vi "Facade.vi"(0 "Data In":T5, 2 "Display State In":T2, 3 "Container State":T4) -> (6 "Data Out":T5, 7 "Display State Out":T2, 8 "Action":T1)   [LabVIEW 2020, in "Input Criterion.xctl"]
uses:
  Input Criterion.xctl
  Data.vi
  Digital Input VIs/Tosca-Input Criterion.ctl
  epl-vi-lib/Utility VIs/Type Defs/Logic State.ctl
  <vilib>/_xctls/Container State.ctl
  State.vi
  Events.ctl
  Event Type.ctl
  Operator.vi
  <vilib>/_xctls/Action.ctl
  <vilib>/_xctls/XControlSupport.lvlib
panel:
  in  "Time":dbl caption="ms"
  in  "Operator":u16(ring) items=["", "AND", "OR"]
  in  "State":u16(ring) caption="for" items=["Low", "High", "Rising", "Falling"]
  in  "Name":u16(ring) caption="is"
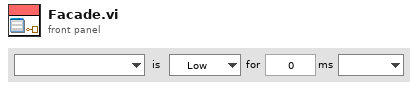
[diagram p1: front panel]
types:
  T1 = typedef "XControlSupport.lvlib/Action.ctl" = cluster{"Data Changed?":bool, "State Changed?":bool, "Action Name":string}
  T2 = typedef "Input Criterion.xctl/State.vi" = cluster{"DI":string[], "Flags":string[], "show op":bool, "flag start":i16, "Events":T3}
  T3 = typedef "Input Criterion.xctl/Events.ctl" = cluster{"Generic":refnum<user-event>, "Operator":refnum<user-event>, "Criterion":refnum<user-event>}
  T4 = typedef "XControlSupport.lvlib/Container State.ctl" = cluster{"Indicator?":bool, "Run Mode?":bool, " Refnum":refnum<vi>}
  T5 = typedef "Input Criterion.xctl/Data.vi" = cluster{"Criterion":T6, "Operator":i16, "visible":bool}
  T6 = typedef "Tosca-Input Criterion.ctl" = cluster{"DigInput":i32, "State":T7, "Time (ms)":i32, "Name":string}
  T7 = typedef "Logic State.ctl" = enum16{"Low", "High", "Rising", "Falling"}
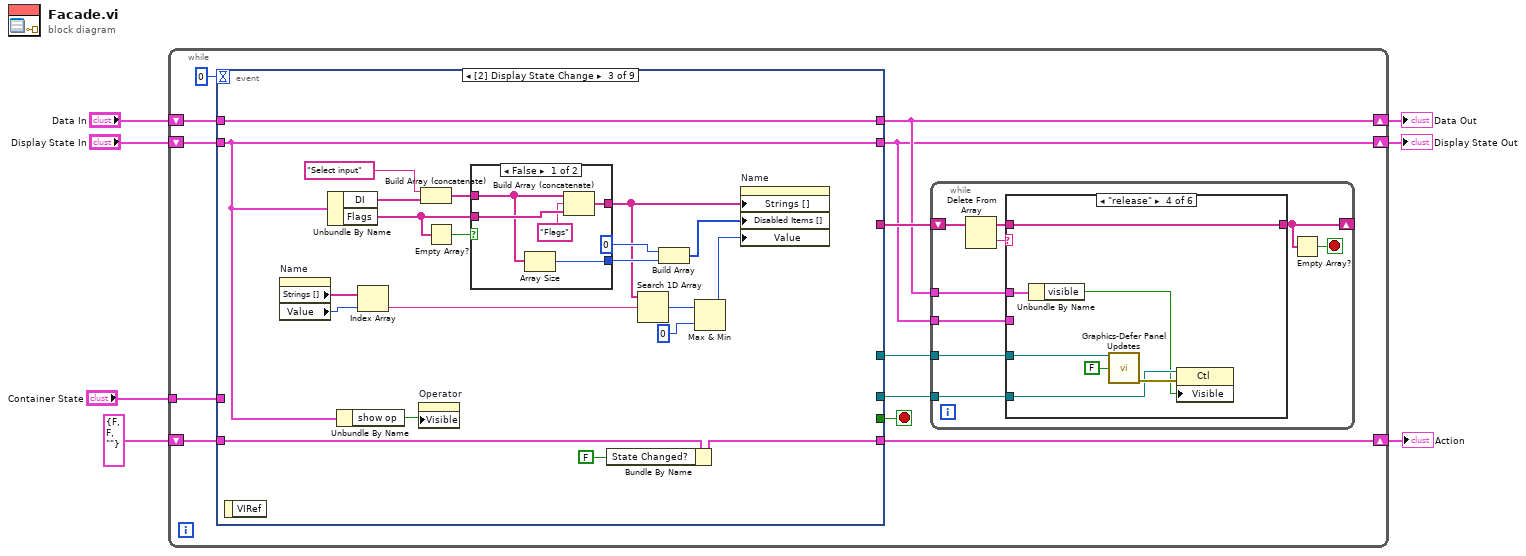
[diagram p0: block diagram]
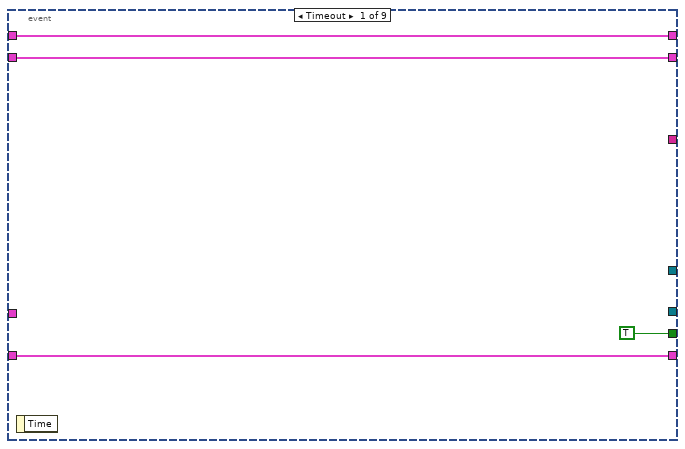
[diagram p2: hidden frame]
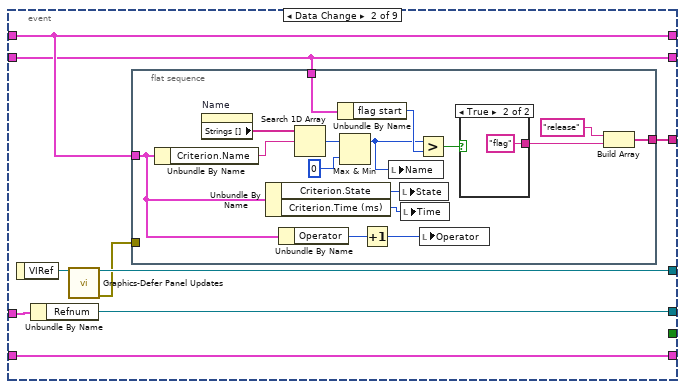
[diagram p3: hidden frame]
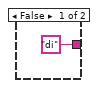
[diagram p4: hidden frame]
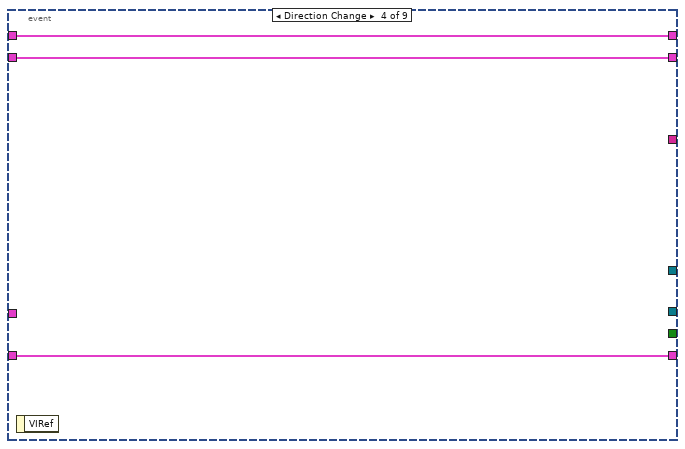
[diagram p6: hidden frame]
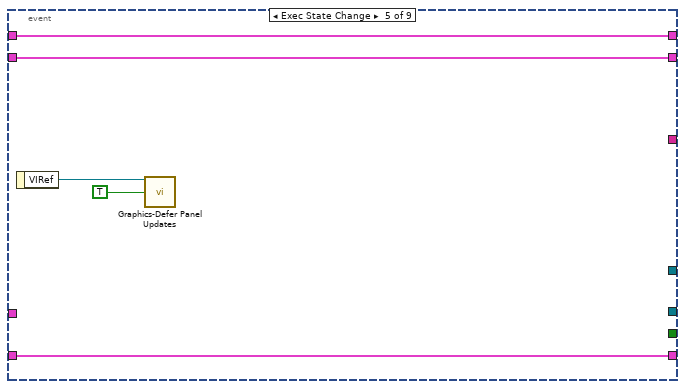
[diagram p7: hidden frame]
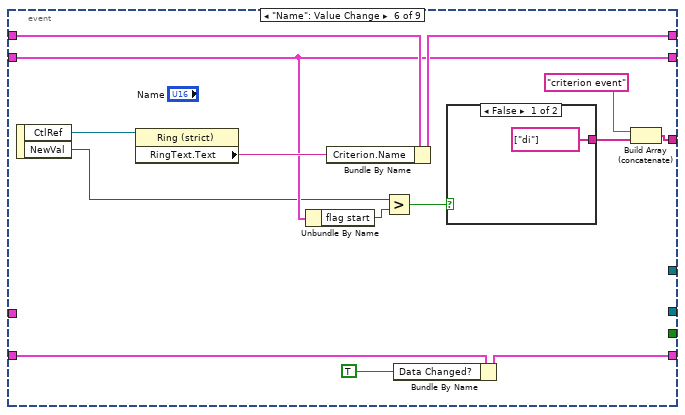
[diagram p8: hidden frame]
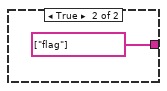
[diagram p9: hidden frame]
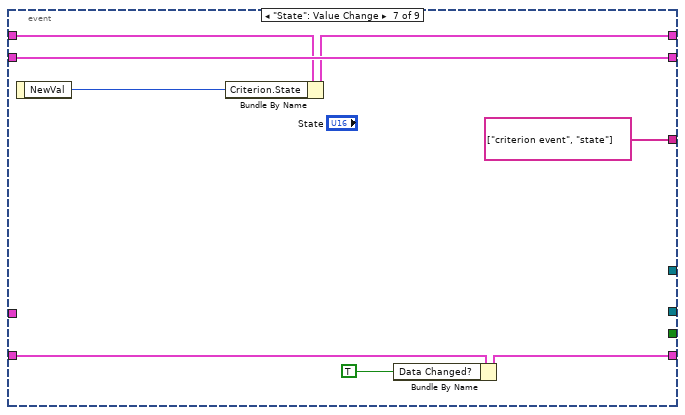
[diagram p10: hidden frame]
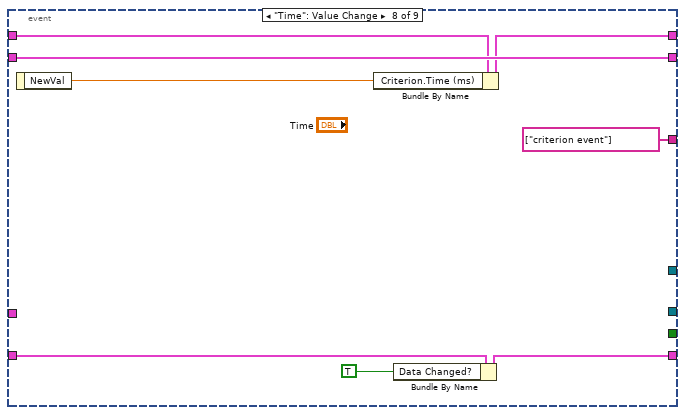
[diagram p11: hidden frame]
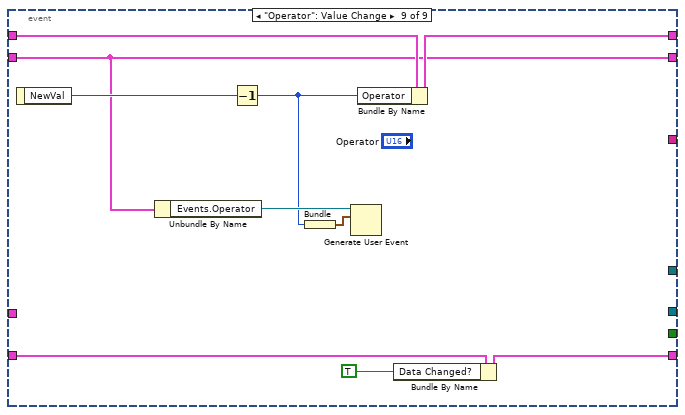
[diagram p12: hidden frame]
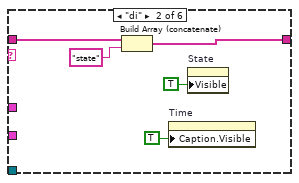
[diagram p14: hidden frame]
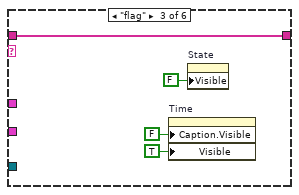
[diagram p15: hidden frame]
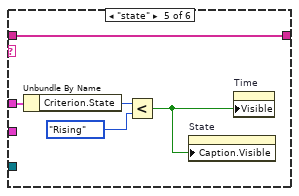
[diagram p16: hidden frame]
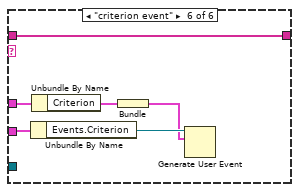
[diagram p17: hidden frame]
diagram:
  n1 = while {
    shift-right: [w9] -> w4
    shift-left: "Display State In" -> [w19]
    tunnel: "Container State" -> [w16]
    shift-right: [w11] -> w7
    shift-left: "Data In" -> [w15]
    shift-right: [w13] -> w2
    shift-left: T1 {"Data Changed?"=FALSE, "State Changed?"=FALSE, "Action Name"=""} ("Action") -> [w14]
    stop <- w18 stop-if-true
    n2 = event shown="[2] Display State Change" {
      selector: _ -> [_ _ _ _ _ _ _ _ _]
      dyn-events: _ -> [_ _ _ _ _ _ _ _ _]
      timeout: 0 -> [_ _ _ _ _ _ _ _ _]
      tunnel: w19 -> [w21 w30 w64 w80 w85 w91 w109 w117 w121]
      tunnel: [w21 w30 w64 w80 w85 w91 w109 w117 w121] -> w9
      tunnel: [TRUE _ _ _ _ _ _ _ _] -> w18
      tunnel: w16 -> [_ w25 _ _ _ _ _ _ _]
      tunnel: w15 -> [w20 w31 w71 w79 w84 w99 w108 w116 w127]
      tunnel: [w20 w31 w71 w79 w84 w94 w103 w112 w123] -> w11
      tunnel: [w22 w32 w60 w78 w83 w97 w106 w114 w125] -> w13
      tunnel: w14 -> [w22 w32 w70 w78 w83 w98 w107 w115 w126]
      tunnel: [_ w29 _ _ _ w87 string[] ["criterion event", "state"] string[] ["criterion event"] _] -> w12
      tunnel: [_ w27 _ _ _ _ _ _ _] -> w10
      tunnel: [_ w24 _ _ _ _ _ _ _] -> w8
      event Timeout {
        n3 = event-data() -> ()  [unwired: 1 in, 1 out]
      }
      event Data Change {
        n4 = event-data() -> ("VIRef"=w28:refnum<vi>)  [unwired: 1 in]
        n5 = Unbundle By Name(w25) -> ("Refnum"=w24:refnum<vi>)
        n6 = call "Graphics-Defer Panel Updates.vi"("VI"=w28) -> ("VI out"=w27:refnum<vi>, "error out"=w26:errorcluster)  [unwired: 13 in]
        n7 = flat-sequence {
          tunnel: w31 -> [w46]
          tunnel: w30 -> [w39]
          tunnel: [w34] -> w29
          tunnel: w26 -> [_]
          frame #0 {
            n8 = Unbundle By Name(w46) -> ("Criterion.Name"=w36:string)
            n9 = property on="Name" class="Ring (strict)"() -> ("Strings []"=w42:string[])  [unwired: 2 in, 2 out]
            n10 = Unbundle By Name(w46) -> ("Criterion.State"=w48:T7, "Criterion.Time (ms)"=w47:i32)
            n11 = Unbundle By Name(w46) -> ("Operator"=w45:i16)
            n12 = Search 1D Array(1D array=w42, element=w36) -> (index of element=w41:i32)  [unwired: 1 in]
            n13 = Unbundle By Name(w39) -> ("flag start"=w38:i16)
            n14 = Max & Min(x=w41, y=0) -> (max(x,y)=w35:i32)  [unwired: 1 out]
            n15 = Increment(x=w45) -> (x+1=w44:i16)
            n16 = local write "Name"(w35) -> ()
            n17 = local write "State"(w48) -> ()
            n18 = local write "Time"(w47) -> ()
            n19 = Greater?(x=w35, y=w38) -> (0:w37:bool)
            n20 = local write "Operator"(w44) -> ()
            n21 = case shown="True" w37 {
              tunnel: ["di" ("String") "flag" ("String")] -> w43
              frame False {
              }
              frame True {
              }
            }
            n22 = Build Array("release" ("element"), w43) -> (w34:string[])
          }
        }
      }
      event Display State Change {
        n23 = event-data() -> ()  [unwired: 1 in, 1 out]
        n24 = property on="Name" class="Ring (strict)"() -> ("Strings []"=w57:string[], "Value"=w56:u16)  [unwired: 2 in, 2 out]
        n25 = Unbundle By Name(w64) -> ("DI"=w69:string[], "Flags"=w65:string[])
        n26 = Unbundle By Name(w64) -> ("show op"=w63:bool)
        n27 = Index Array(array=w57, index=w56) -> (element=w54:string)
        n28 = property on="Operator" class="Ring (strict)"("Visible"=w63) -> ()  [unwired: 2 in, 2 out]
        n29 = Build Array (concatenate)("Select input", w69) -> (w67:string[])
        n30 = Empty Array?(array=w65) -> (empty?=w66:bool)
        n31 = case shown="False" w66 {
          tunnel: w67 -> [w73 w77]
          tunnel: w65 -> [w76 _]
          tunnel: [w74 w77] -> w55
          tunnel: [w72 _] -> w58
          frame False {
            n32 = Array Size(array=w73) -> (size(s)=w72:i32)
            n33 = Build Array (concatenate)(w73, "Flags", w76) -> (w74:string[])
          }
          frame True {
          }
        }
        n34 = Bundle By Name(cluster=w70, "State Changed?"=FALSE) -> (w60:T1)
        n35 = Search 1D Array(1D array=w55, element=w54) -> (index of element=w53:i32)  [unwired: 1 in]
        n36 = Build Array(0, w58) -> (w62:i32[])
        n37 = Max & Min(x=w53, y=0) -> (max(x,y)=w52:i32)  [unwired: 1 out]
        n38 = property on="Name" class="Ring (strict)"("Strings []"=w55, "Disabled Items []"=w62, "Value"=w52) -> ()  [unwired: 2 in, 2 out]
      }
      event Direction Change {
        n39 = event-data() -> ()  [unwired: 1 in, 1 out]
      }
      event Exec State Change {
        n40 = event-data() -> ("VIRef"=w82:refnum<vi>)  [unwired: 1 in]
        n41 = call "Graphics-Defer Panel Updates.vi"("VI"=w82, "Defer (F)"=TRUE) -> ()  [unwired: 12 in, 2 out]
      }
      event "Name": Value Change {
        n42 = event-data() -> ("CtlRef"=w93:refnum<vi>, "NewVal"=w90:u16)  [unwired: 1 in]
        n43 = property class="Ring (strict)"(reference=w93) -> ("RingText.Text"=w92:string)  [unwired: 1 in, 2 out]
        n44 = Unbundle By Name(w91) -> ("flag start"=w89:i16)
        n45 = Bundle By Name(cluster=w99, "Criterion.Name"=w92) -> (w94:T5)
        n46 = Greater?(x=w90, y=w89) -> (0:w88:bool)
        n47 = Bundle By Name(cluster=w98, "Data Changed?"=TRUE) -> (w97:T1)
        n48 = case shown="False" w88 {
          tunnel: [string[] ["di"] string[] ["flag"]] -> w95
          frame False {
          }
          frame True {
          }
        }
        n49 = Build Array (concatenate)("criterion event", w95) -> (w87:string[])
      }
      event "State": Value Change {
        n50 = event-data() -> ("NewVal"=w102:u16)  [unwired: 1 in]
        n51 = Bundle By Name(cluster=w108, "Criterion.State"=w102) -> (w103:T5)
        n52 = Bundle By Name(cluster=w107, "Data Changed?"=TRUE) -> (w106:T1)
      }
      event "Time": Value Change {
        n53 = event-data() -> ("NewVal"=w111:dbl)  [unwired: 1 in]
        n54 = Bundle By Name(cluster=w116, "Criterion.Time (ms)"=w111) -> (w112:T5)
        n55 = Bundle By Name(cluster=w115, "Data Changed?"=TRUE) -> (w114:T1)
      }
      event "Operator": Value Change {
        n56 = event-data() -> ("NewVal"=w122:u16)  [unwired: 1 in]
        n57 = Unbundle By Name(w121) -> ("Events.Operator"=w120:refnum<user-event>)
        n58 = Decrement(x=w122) -> (x-1=w119:u16)
        n59 = Bundle(w119) -> (w118:cluster{u16})  [unwired: 1 in]
        n60 = Generate User Event(user event=w120, event data cluster=w118) -> ()  [unwired: 2 in, 2 out]
        n61 = Bundle By Name(cluster=w127, "Operator"=w119) -> (w123:T5)
        n62 = Bundle By Name(cluster=w126, "Data Changed?"=TRUE) -> (w125:T1)
      }
    }
    n63 = while {
      shift-right: [w133] -> _
      shift-left: w12 -> [w136]
      tunnel: w11 -> [w131]
      tunnel: w10 -> [w130]
      tunnel: w9 -> [w129]
      tunnel: w8 -> [w128]
      stop <- w132 stop-if-true
      n64 = Delete From Array(array=w136) -> (deleted portion=w134:string, array with subset deleted=w135:string[])  [unwired: 2 in]
      n65 = case shown="\"release\"" w134 {
        tunnel: w135 -> [w137 w142 w146 w153 w158 w164]
        tunnel: [w137 w139 w146 w153 w158 w164] -> w133
        tunnel: w131 -> [_ _ _ w148 w157 w162]
        tunnel: w130 -> [_ _ _ w151 _ _]
        tunnel: w129 -> [_ _ _ _ _ w163]
        tunnel: w128 -> [_ _ _ w149 _ _]
        frame "", Default {
        }
        frame "di" {
          n66 = Build Array (concatenate)(w142, "state") -> (w139:string[])
          n67 = property on="Time" class="DigNum (strict)"("Caption.Visible"=TRUE) -> ()  [unwired: 2 in, 2 out]
          n68 = property on="State" class="Ring (strict)"("Visible"=TRUE) -> ()  [unwired: 2 in, 2 out]
        }
        frame "flag" {
          n69 = property on="Time" class="DigNum (strict)"("Caption.Visible"=FALSE, "Visible"=TRUE) -> ()  [unwired: 2 in, 2 out]
          n70 = property on="State" class="Ring (strict)"("Visible"=FALSE) -> ()  [unwired: 2 in, 2 out]
        }
        frame "release" {
          n71 = Unbundle By Name(w148) -> ("visible"=w147:bool)
          n72 = call "Graphics-Defer Panel Updates.vi"("VI"=w151, "Defer (F)"=FALSE) -> ("error out"=w150:errorcluster)  [unwired: 12 in, 1 out]
          n73 = property class="Ctl"(reference=w149, error in=w150, "Visible"=w147) -> ()  [unwired: 2 out]
        }
        frame "state" {
          n74 = Unbundle By Name(w157) -> ("Criterion.State"=w156:T7)
          n75 = Less?(x=w156, y=Logic_State."Rising") -> (x < y?=w154:bool)
          n76 = property on="State" class="Ring (strict)"("Caption.Visible"=w154) -> ()  [unwired: 2 in, 2 out]
          n77 = property on="Time" class="DigNum (strict)"("Visible"=w154) -> ()  [unwired: 2 in, 2 out]
        }
        frame "criterion event" {
          n78 = Unbundle By Name(w163) -> ("Events.Criterion"=w160:refnum<user-event>)
          n79 = Unbundle By Name(w162) -> ("Criterion"=w161:T6)
          n80 = Bundle("Criterion"=w161) -> (w159:cluster{"Criterion":T6})  [unwired: 1 in]
          n81 = Generate User Event(user event=w160, event data cluster=w159) -> ()  [unwired: 2 in, 2 out]
        }
      }
      n82 = Empty Array?(array=w133) -> (empty?=w132:bool)
    }
  }
  "Display State Out" <- w4
  "Data Out" <- w7
  "Action" <- w2
